vi "GetIndicatorTermIdx.vi"(11 "BaseAccessorScripter in":refnum<class "BaseAccessorScripter.lvclass">) -> (2 "TermIdx":u32=2, 3 "BaseAccessorScripter out":refnum<class "BaseAccessorScripter.lvclass">)   [LabVIEW 2021, in "MemberVICreation.lvlib" / "BaseAccessorScripter.lvclass"]
uses:
  <resource>/Framework/Providers/LVClassLibrary/NewAccessors/BaseAccessorScripter/BaseAccessorScripter.lvclass
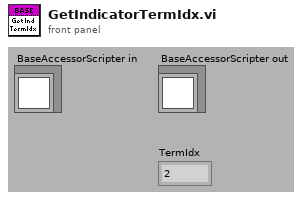
[diagram p1: front panel]
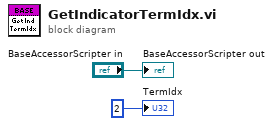
[diagram p0: block diagram]
diagram:
  "BaseAccessorScripter out" <- "BaseAccessorScripter in"
  "TermIdx" <- u32 2 ("TermIdx")
